vi "ShowRange v0.2.vi"(2 "Current Grating Density":enum16{"150", "300", "600", "1200", "1800"}(ring)=enum."600" caption="Grating Density", 3 "Central Wavelength":dbl=600.0 caption="nm" format="%.4f") -> (0 "Final Grating Density":enum16{"150", "300", "600", "1200", "1800"}(ring)=enum."600" caption="Current", 1 "CWL buffer":dbl=600.0 caption="Final Center Wavelength" format="%.2f")   [LabVIEW 2021]
doc: "Creates an X-axis for a CCD camera. \nNo global variables is used.\n\nUnit: 0:nm, 1:cm-1, 2:meV"
panel:
  in  "Return":bool=TRUE
  out "meV buffer":dbl=2066.4040666666665 format="%.2f"
  out "cm-1 buffer":dbl=16666.666666666668 format="%.2f"
  in  "Central cm-1":dbl=16666.666666666668 caption="cm-1" format="%.2f"
  in  "Central meV":dbl=2066.4040666666665 caption="meV" format="%.3f"
  out "Emax (cm-1)":dbl=57.29490371241775 format="%.4f"
  out "Emax (cm-1)":dbl=1595.705715333208 format="%.2f"
  out "Emax (meV)":dbl=197.8423661020638 format="%.2f"
  out "Emax (cm-1)":dbl=571.2504622529284 format="%.4f"
  out "Emin (cm-1":dbl=628.5453659653462 format="%.4f"
  out "Emax (cm-1)":dbl=17505.45629418217 format="%.2f"
  out "Emin (cm-1":dbl=15909.750578848963 format="%.2f"
  out "Emax (meV)":dbl=2170.4007572687524 format="%.2f"
  out "Emin (meV)":dbl=1972.5583911666886 format="%.2f"
  out "Spectrometer Focal length":dbl=750.0 format="%.1f"
  out "Detector Pixel Distance":dbl=27.0 format="%.2f"
  out "beta":dbl=0.03851514953863218 format="%.2f"
  out "alpha":dbl=21.141484850461367 format="%.2f"
  out "Spectrometer Mirror angle":dbl=21.18 format="%.2f"
  # "mm"
  # "degrees"
  # "mm"
  # "Parameters of Spectrometer System"
  # "gr/mm"
  # "Center Position"
  # "Min"
  # "Max"
  # "D"
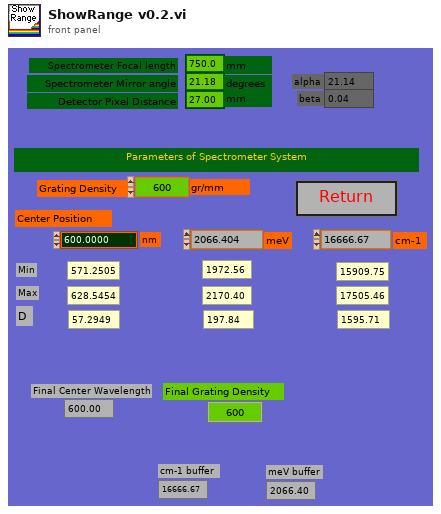
[diagram p1: front panel]
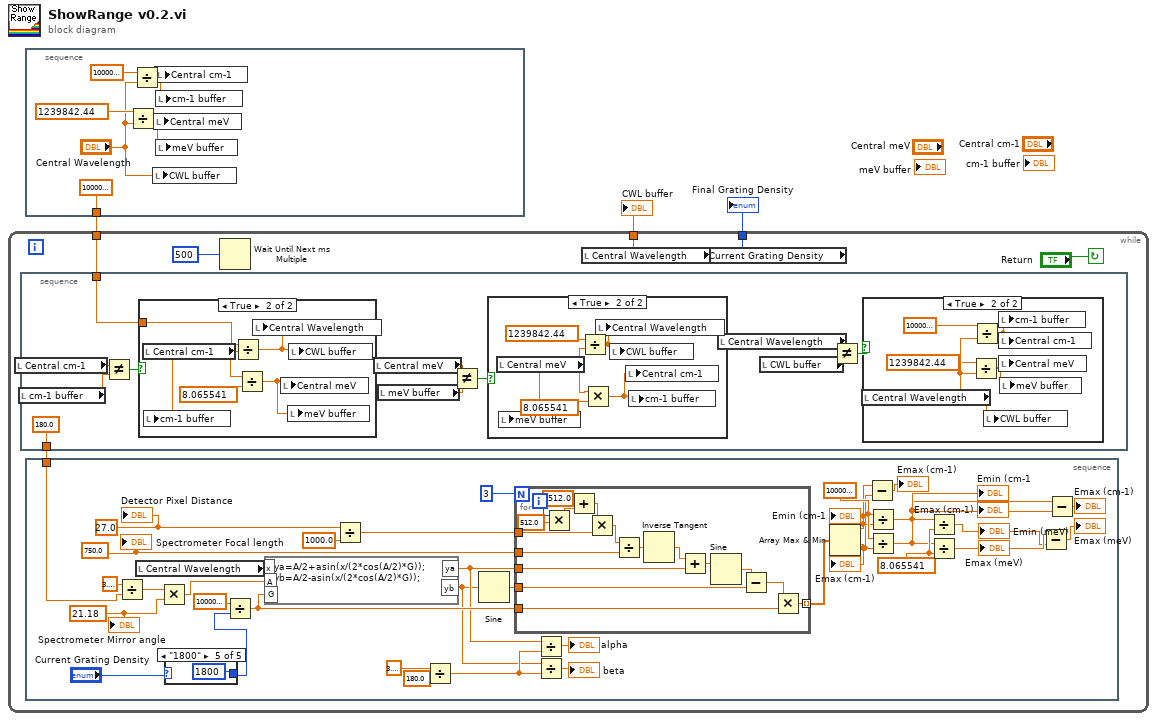
[diagram p0: block diagram]
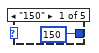
[diagram p5: hidden frame]
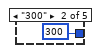
[diagram p6: hidden frame]
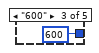
[diagram p7: hidden frame]
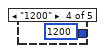
[diagram p8: hidden frame]
diagram:
  n1 = stacked-sequence {
    tunnel: [10000000.0 ("x")] -> w3
    frame #0 {
      n2 = Divide(x=1239842.44, y="Central Wavelength") -> (x/y=w6:dbl)
      n3 = Divide(x=10000000.0, y="Central Wavelength") -> (x/y=w5:dbl)
      n4 = local write "CWL buffer"("Central Wavelength") -> ()
      n5 = local write "Central meV"(w6) -> ()
      n6 = local write "Central cm-1"(w5) -> ()
      n7 = local write "cm-1 buffer"(w5) -> ()
      n8 = local write "meV buffer"(w6) -> ()
    }
  }
  n9 = while {
    tunnel: [w10] -> w1
    tunnel: [w11] -> w2
    tunnel: w3 -> [w12]
    stop <- "Return" continue-if-true
    n10 = stacked-sequence {
      tunnel: [180.0] -> w13
      tunnel: w12 -> [w16]
      frame #0 {
        n11 = local read "Central cm-1"() -> (w20:dbl)
        n12 = local read "cm-1 buffer"() -> (w19:dbl)
        n13 = Not Equal?(x=w20, y=w19) -> (x != y?=w18:bool)
        n14 = case shown="True" w18 {
          tunnel: w16 -> [_ w27]
          frame False {
          }
          frame True {
            n15 = local read "Central cm-1"() -> (w30:dbl)
            n16 = local write "cm-1 buffer"(w30) -> ()
            n17 = Divide(x=w27, y=w30) -> (x/y=w31:dbl)
            n18 = Divide(x=w30, y=8.065541) -> (x/y=w28:dbl)
            n19 = local write "Central Wavelength"(w31) -> ()
            n20 = local write "Central meV"(w28) -> ()
            n21 = local write "meV buffer"(w28) -> ()
            n22 = local write "CWL buffer"(w31) -> ()
          }
        }
        n23 = local read "Central meV"() -> (w23:dbl)
        n24 = local read "meV buffer"() -> (w22:dbl)
        n25 = Not Equal?(x=w23, y=w22) -> (x != y?=w21:bool)
        n26 = case shown="True" w21 {
          frame False {
          }
          frame True {
            n27 = local read "Central meV"() -> (w35:dbl)
            n28 = local write "meV buffer"(w35) -> ()
            n29 = Divide(x=1239842.44, y=w35) -> (x/y=w32:dbl)
            n30 = Multiply(x=w35, y=8.065541) -> (x*y=w33:dbl)
            n31 = local write "Central Wavelength"(w32) -> ()
            n32 = local write "CWL buffer"(w32) -> ()
            n33 = local write "Central cm-1"(w33) -> ()
            n34 = local write "cm-1 buffer"(w33) -> ()
          }
        }
        n35 = local read "Central Wavelength"() -> (w26:dbl)
        n36 = local read "CWL buffer"() -> (w25:dbl)
        n37 = Not Equal?(x=w26, y=w25) -> (x != y?=w24:bool)
        n38 = case shown="True" w24 {
          frame False {
          }
          frame True {
            n39 = local read "Central Wavelength"() -> (w41:dbl)
            n40 = Divide(x=1239842.44, y=w41) -> (x/y=w38:dbl)
            n41 = Divide(x=10000000.0, y=w41) -> (x/y=w37:dbl)
            n42 = local write "CWL buffer"(w41) -> ()
            n43 = local write "cm-1 buffer"(w37) -> ()
            n44 = local write "Central cm-1"(w37) -> ()
            n45 = local write "Central meV"(w38) -> ()
            n46 = local write "meV buffer"(w38) -> ()
          }
        }
      }
    }
    n47 = stacked-sequence {
      tunnel: w13 -> [w44]
      frame #0 {
        w57 = 21.18 ("Detector Pixel Distance")
        w56 = 750.0 ("Detector Pixel Distance")
        w58 = 27.0 ("x")
        w69 = 8.065541
        w70 = 10000000.0
        n48 = Divide(x=3.141592653589793, y=w44) -> (x/y=w50:dbl)
        n49 = local read "Central Wavelength"() -> (w46:dbl)
        n50 = Multiply(x=w50, y=w57) -> (x*y=w55:dbl)
        n51 = case shown="\"1800\"" "Current Grating Density" {
          tunnel: [150 300 600 1200 1800] -> w42
          frame "150" {
          }
          frame "300" {
          }
          frame "600" {
          }
          frame "1200" {
          }
          frame "1800" {
          }
        }
        n52 = Divide(x=1000000.0, y=w42) -> (x/y=w54:dbl)
        n53 = formula code="ya=A/2+asin(x/(2*cos(A/2)*G));\nyb=A/2-asin(x/(2*cos(A/2)*G));"("x"=w46, "A"=w55, "G"=w54) -> ("ya"=w48:dbl, "yb"=w47:dbl)
        n54 = Divide(x=w58, y=1000.0) -> (x/y=w72:dbl)
        n55 = Divide(x=3.141592653589793, y=180.0) -> (x/y=w53:dbl)
        n56 = Sine(x=w47) -> (sin(x)=w71:dbl)
        n57 = for {
          N: 3 -> [_]
          tunnel: w56 -> [w96]
          tunnel: w72 -> [w85]
          tunnel: w71 -> [w94]
          tunnel: [w92] -> w59 mode=indexing
          tunnel: w54 -> [w91]
          tunnel: w48 -> [w86]
          i -> [w98]
          n58 = Multiply(x=w98, y=512.0) -> (x*y=w83:dbl)
          n59 = Add(x=-512.0, y=w83) -> (x+y=w82:dbl)
          n60 = Multiply(x=w82, y=w85) -> (x*y=w87:dbl)
          n61 = Divide(x=w87, y=w96) -> (x/y=w90:dbl)
          n62 = Inverse Tangent(1:w90) -> (0:w89:dbl)
          n63 = Add(x=w89, y=w86) -> (x+y=w88:dbl)
          n64 = Sine(x=w88) -> (sin(x)=w95:dbl)
          n65 = Subtract(x=w95, y=w94) -> (x-y=w93:dbl)
          n66 = Multiply(x=w93, y=w91) -> (x*y=w92:dbl)
        }
        n67 = Divide(x=w48, y=w53) -> (x/y=→"alpha":dbl)
        n68 = Divide(x=w47, y=w53) -> (x/y=→"beta":dbl)
        n69 = Array Max & Min(array=w59) -> (max value=w63:dbl, min value=w62:dbl)  [unwired: 2 out]
        "Emin (cm-1" <- w63
        "Emax (cm-1)" <- w62
        n70 = Subtract(x=w63, y=w62) -> (x-y=→"Emax (cm-1)":dbl)
        n71 = Divide(x=w70, y=w63) -> (x/y=w67:dbl)
        "Emin (cm-1" <- w67
        n72 = Divide(x=w70, y=w62) -> (x/y=w66:dbl)
        "Emax (cm-1)" <- w66
        n73 = Divide(x=w67, y=w69) -> (x/y=w65:dbl)
        "Emin (meV)" <- w65
        n74 = Divide(x=w66, y=w69) -> (x/y=w68:dbl)
        "Emax (meV)" <- w68
        n75 = Subtract(x=w68, y=w65) -> (x-y=→"Emax (meV)":dbl)
        n76 = Subtract(x=w66, y=w67) -> (x-y=→"Emax (cm-1)":dbl)
        "Spectrometer Focal length" <- w56
        "Spectrometer Mirror angle" <- w57
        "Detector Pixel Distance" <- w58
      }
    }
    n77 = Wait Until Next ms Multiple(millisecond multiple=u32 500) -> ()  [unwired: 1 out]
    n78 = local read "Central Wavelength"() -> (w11:dbl)
    n79 = local read "Current Grating Density"() -> (w10:enum16{"150", "300", "600", "1200", "1800"})
  }
  "CWL buffer" <- w2
  "Final Grating Density" <- w1
